vi "Our Mecanum Drive.vi"(7 "Max Output":dbl, 8 "Gyro Angle":dbl, 9 "X":dbl, 10 "Y":dbl, 11 "Rotation":dbl) -> (0 "Rear Right":dbl, 1 "Rear Left":dbl, 2 "Front Right":dbl, 3 "Front Left":dbl)   [LabVIEW 2014]
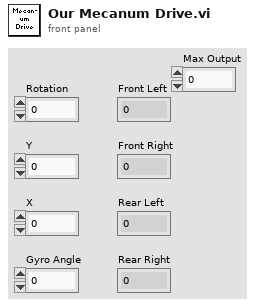
[diagram p1: front panel]
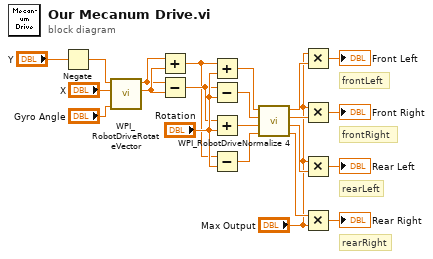
[diagram p0: block diagram]
diagram:
  # "rearLeft"
  # "frontRight"
  # "rearRight"
  # "frontLeft"
  n1 = Negate(x="Y") -> (-x=w22:dbl)
  n2 = call <vilib>:"WPI_RobotDriveRotateVector.vi"("Angle"="Gyro Angle", "X"="X", "Y"=w22) -> ("X'"=w8:dbl, "Y'"=w7:dbl)  [unwired: 7 out]
  n3 = Add(x=w7, y=w8) -> (x+y=w10:dbl)
  n4 = Subtract(x=w7, y=w8) -> (x-y=w12:dbl)
  n5 = Add(x=w10, y="Rotation") -> (x+y=w14:dbl)
  n6 = Subtract(x=w12, y="Rotation") -> (x-y=w13:dbl)
  n7 = Add(x=w12, y="Rotation") -> (x+y=w11:dbl)
  n8 = Subtract(x=w10, y="Rotation") -> (x-y=w9:dbl)
  n9 = call <vilib>:"WPI_RobotDriveNormalize 4.vi"("D"=w9, "C"=w11, "B"=w13, "A"=w14) -> ("D'"=w18:dbl, "C'"=w19:dbl, "B'"=w17:dbl, "A'"=w6:dbl)
  n10 = Multiply(x="Max Output", y=w6) -> (x*y=→"Front Left":dbl)
  n11 = Multiply(x="Max Output", y=w17) -> (x*y=→"Front Right":dbl)
  n12 = Multiply(x="Max Output", y=w19) -> (x*y=→"Rear Left":dbl)
  n13 = Multiply(x=w18, y="Max Output") -> (x*y=→"Rear Right":dbl)
